vi "test_Determine Trigger_Expected outputs if Generation Type is Trigger Only.vi"(8 "error in (no error)":errorcluster, 11 "TestCase in":refnum<class "Instrument Addon Unit Tests.lvclass">) -> (0 "error out":errorcluster, 3 "TestCase out":refnum<class "Instrument Addon Unit Tests.lvclass">)   [LabVIEW 2020, in "Instrument Addon Unit Tests.lvclass"]
uses:
  Instrument Addon Unit Tests.lvclass
  Addon/Addon Shared/Types/Command Channel Indeces.ctl
  Addon/Addon Shared/Types/Command Channel Index.ctl
  Addon/Addon Shared/Types/Message Parameters.ctl
  Addon/Addon Shared/Types/Message Generation Type.ctl
  <vilib>/addons/_JKI Toolkits/VI Tester/TestCase.llb/TestCase.lvclass
  Addon/Addon Engine/Instrument Addon Engine.lvlib
  Addon/Addon Shared/Instrument Addon Shared.lvlib
  C:/Program Files (x86)/National Instruments/LabVIEW 2020/vi.lib/addons/_JKI Toolkits/VI Tester/TestCase.llb/TestCase.lvclass
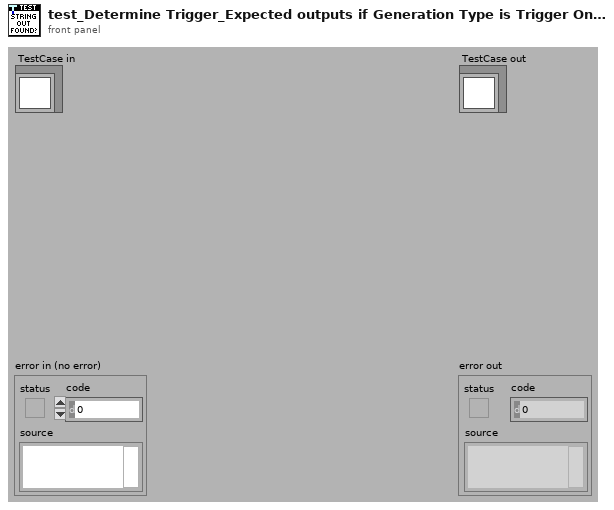
[diagram p1: front panel]
types:
  T1 = typedef "Instrument Addon Shared.lvlib/Command Channel Indeces.ctl" = cluster{"Channels":T2[]}
  T2 = typedef "Instrument Addon Shared.lvlib/Command Channel Index.ctl" = cluster{"Data Index":i32, "Data Length":i32}
  T3 = typedef "Instrument Addon Shared.lvlib/Message Parameters.ctl" = cluster{"Generation Type":T4, "Period":dbl, "Include Protection":bool, "Type":string}
  T4 = typedef "Instrument Addon Shared.lvlib/Message Generation Type.ctl" = enum16{"Trigger Only", "Periodic & Trigger", "Value Change & Trigger"}
  T5 = cluster{"Trigger":bool, "Command Indeces":T1, "Detect?":bool[], "Enabled":i32, "Time Since Last Generation":u32, "Message Parameters":T3}
  T6 = cluster{"Trigger":bool, "Time Since Last Generation":u32}
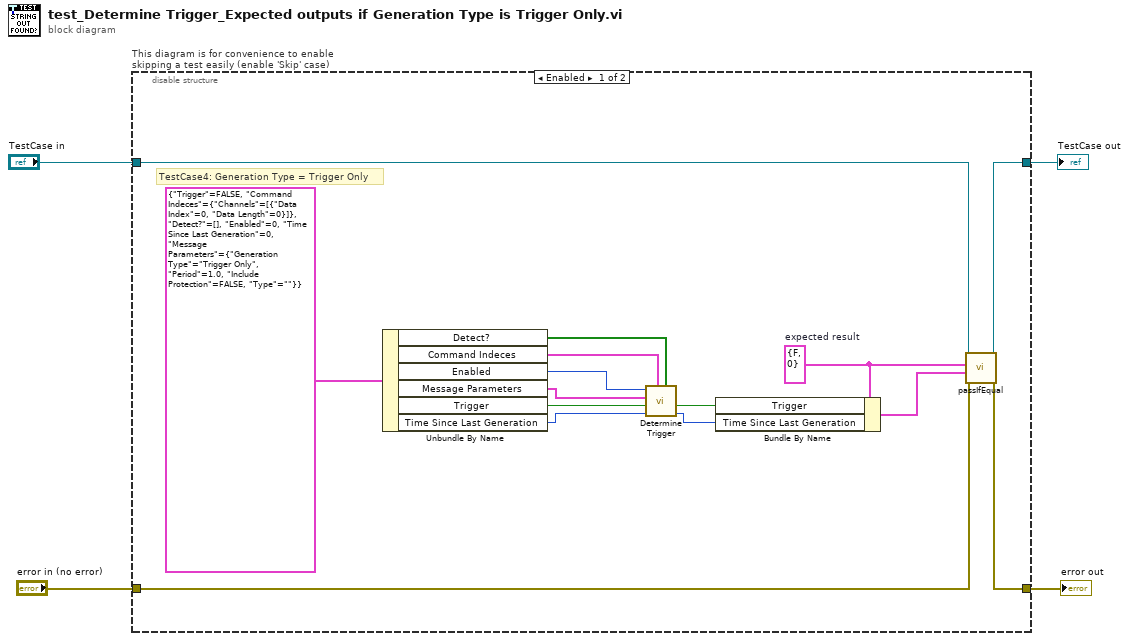
[diagram p0: block diagram]
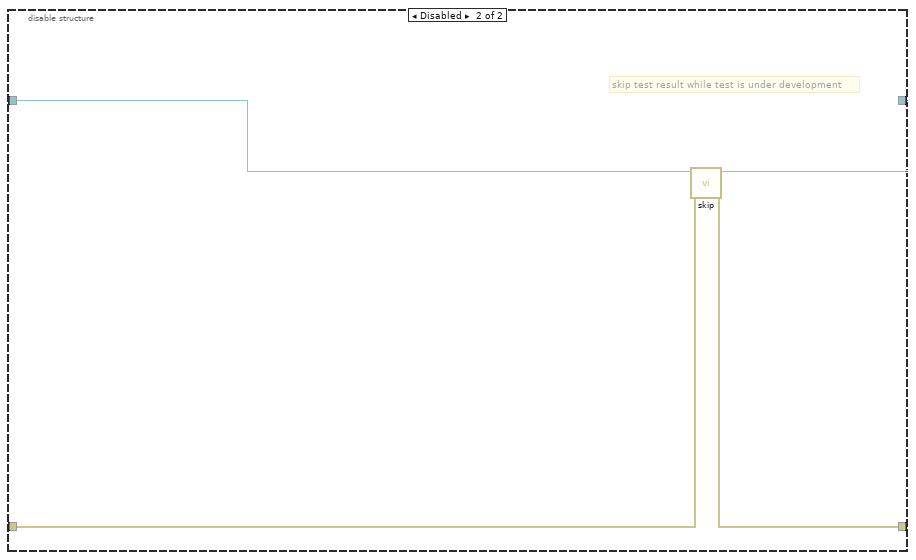
[diagram p2: hidden frame]
diagram:
  n1 = disable-structure "This diagram is for convenience to enable skipping a test easily (enable 'Skip' case)" shown="Enabled" {
    disable-tunnel: "TestCase in" -> [w17 w23]
    disable-tunnel: [w18 w21] -> w1
    disable-tunnel: [w19 w22] -> w3
    disable-tunnel: "error in (no error)" -> [w16 w20]
    frame Enabled {
      w11 = T6 {"Trigger"=FALSE, "Time Since Last Generation"=0}  # expected result
      # "TestCase4: Generation Type = Trigger Only"
      n2 = Unbundle By Name(T5 {"Trigger"=FALSE, "Command Indeces"={"Channels"=[{"Data Index"=0, "Data Length"=0}]}, "Detect?"=[], "Enabled"=0, "Time Since Last Generation"=0, "Message Parameters"={"Generation Type"=enum."Trigger Only", "Period"=1.0, "Include Protection"=FALSE, "Type"=""}}) -> ("Detect?"=w15:bool[], "Command Indeces"=w14:T1, "Enabled"=w10:i32, "Message Parameters"=w13:T3, "Trigger"=w12:bool, "Time Since Last Generation"=w7:u32)
      n3 = call "Determine Trigger.vi"("Detect?"=w15, "Command Indeces"=w14, "Time Since Last Generation"=w7, "Trigger"=w12, "Message Parameters"=w13, "Enabled"=w10) -> ("Time Since Last Generation"=w8:u32, "Trigger"=w9:bool)  [unwired: 4 in]
      n4 = Bundle By Name(cluster=w11, "Trigger"=w9, "Time Since Last Generation"=w8) -> (w6:T6)
      n5 = call-dynamic "passIfEqual.vi"("error in (no error)"=w16, "y"=w6, "x"=w11, "TestCase in"=w17) -> ("error out"=w19:errorcluster, "TestCase out"=w18:refnum<class "Instrument Addon Unit Tests.lvclass">)  [unwired: 6 in]
    }
    frame Disabled {
      # "skip test result while test is under development"
      n6 = call <vilib>:"skip.vi"("error in (no error)"=w20, "TestCase in"=w23) -> ("error out"=w22:errorcluster, "TestCase out"=w21:refnum<class "Instrument Addon Unit Tests.lvclass">)  [unwired: 8 in]
    }
  }
  "error out" <- w3
  "TestCase out" <- w1
